vi "Demo.vi"() -> ()   [LabVIEW 2021, in "Context Actor.lvlib" / "Context Actor.lvclass"]
uses:
  Context Actor.lvclass
  A Context State/A Context State.lvclass
  C:/PPLs/Design-Patterns/State Pattern/Context Actor/Context State/Context State.lvclass
  B Context State/B Context State.lvclass
  C:/PPLs/Design-Patterns/State Pattern/State Pattern/State Pattern.lvclass
  Context Actor.lvclass/Context Actor.ctl
  State Pattern/State Pattern.lvclass
panel:
  out "Context I32 2":i32
  out "Context I32 1":i32
  # "Overview: Demonstrates the use of State Pattern using composition and AF messages. Context.lvlib is an Actor library that uses the state pattern. Composed State Pattern.lvlib is the library used to aid in developing the state pattern, with precreated State Transition.vi message along with logic to determine if a state may be transitioned into. All classes have unique colors and corresponding colored wires. This makes for easily seeing which common parent class exists on the block diagram.\n\nInstructions:\n1. View -> Bookmark Manager. Open the three #Demo bookmarks, keep their front panels open. Close their block diagrams.\n2. Before running this VI, note that the first state is transitioned into (Numeric) here using the State Transition.vi before Launch Root Actor. Subsequent state transitions occur by use of the front panel buttons. The states below implement that state transition. Closing the front panel Exits the current state.\n3. State messages are executed by use of the front panel buttons. The states below implement that message.\n2. Run this VI."
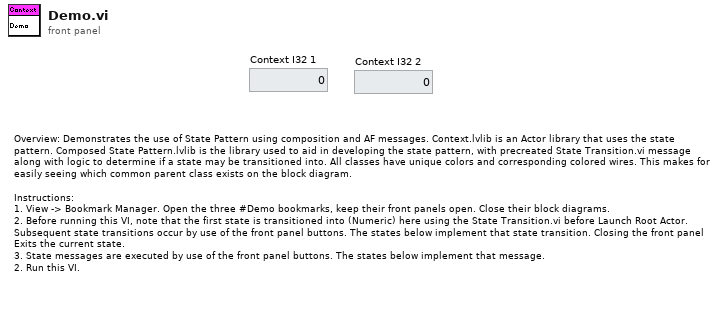
[diagram p1: front panel]
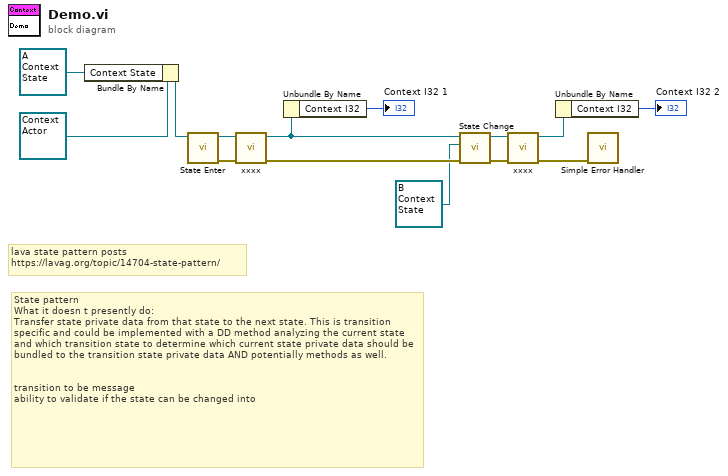
[diagram p0: block diagram]
diagram:
  # "State pattern\nWhat it doesn t presently do:\nTransfer state private data from that state to the next state. This is transition specific and could be implemented with a DD method analyzing the current state and which transition state to determine which current state private data should be bundled to the transition state private data AND potentially methods as well.\n\n\ntransition to be message\nability to validate if the state can be changed into"
  # "lava state pattern posts\nhttps://lavag.org/topic/14704-state-pattern/"
  n1 = Bundle By Name(cluster=refnum<class "Context Actor.lvclass"> refnum ("Context Actor.lvlib:Context Actor.lvclass"), "Context State"=refnum<class "A Context State.lvclass"> refnum ("A Context State.lvclass")) -> (w11:refnum<class "Context Actor.lvclass">)
  n2 = call "State Enter.vi"("State Pattern in"=w11) -> ("error out"=w8:errorcluster, "State Pattern out"=w10:refnum<class "Context Actor.lvclass">)  [unwired: 9 in]
  n3 = call-dynamic "xxxx.vi"("error in (no error)"=w8, "Context Actor in"=w10) -> ("error out"=w7:errorcluster, "Context Actor out"=w9:refnum<class "Context Actor.lvclass">)  [unwired: 8 in]
  n4 = Unbundle By Name(w9) -> ("Context I32"=→"Context I32 1":i32)
  n5 = call "State Change.vi"("error in"=w7, "Transition State"=refnum<class "B Context State.lvclass"> refnum ("B Context State.lvclass"), "State Pattern in"=w9) -> ("error out"=w3:errorcluster, "State Pattern out"=w5:refnum<class "Context Actor.lvclass">)  [unwired: 7 in]
  n6 = call-dynamic "xxxx.vi"("error in (no error)"=w3, "Context Actor in"=w5) -> ("error out"=w2:errorcluster, "Context Actor out"=w4:refnum<class "Context Actor.lvclass">)  [unwired: 8 in]
  n7 = Unbundle By Name(w4) -> ("Context I32"=→"Context I32 2":i32)
  n8 = call <vilib>:"Simple Error Handler.vi"("error in (no error)"=w2) -> ()  [unwired: 4 in, 5 out]
